vi "Get property names from config.vi"(0 "reference in":refnum<class "metadata.lvclass">, 5 "error in (no error)":errorcluster) -> (10 "section names":string[](array[string]), 14 "reference out":refnum<class "metadata.lvclass">, 15 "nb elements":u16, 16 "Property names []":string[](array[string]), 19 "error out":errorcluster)   [LabVIEW 2019, in "metadata.lvclass"]
uses:
  metadata.lvclass
  <vilib>/Utility/config.llb/NI_LVConfig.lvlib
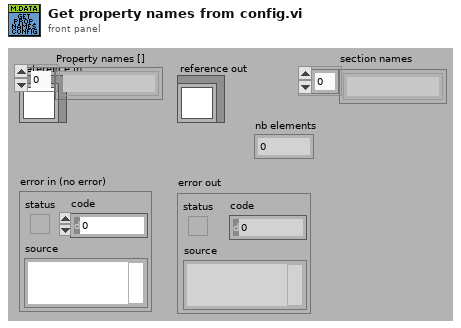
[diagram p1: front panel]
types:
  T1 = typedef "metadata.lvclass/ObjectAttributesRef.ctl" = refnum<data-value>
  T2 = typedef "metadata.lvclass/ObjectAttributes.ctl" = cluster{"MyAttribute":dbl, "System Control":T3, "file info":T4, "Sample info":T5, "Cantilever info":T6, "XYZ piezos":T7, "Mapping":T8, "Fcurve segment":T9[], "Fast fpga segment":T11, "Chirp":T12, "precision (6)":i16, "width (-)":i16, "Metadata":T13, "config filepath":path, "Section names []":string[], "Property names []":string[], "nb elements":u16}
  T3 = typedef "metadata.lvclass/System control parameters.ctl" = cluster{"FPGA SW version":string, "TDMS file version":string, "Instrument":string, "Instrument model":string, "Instrument scanner":string, "Instrument clockrate (Mhz)":string, "Instrument tick time (us)":string}
  T4 = typedef "metadata.lvclass/File info parameters.ctl" = cluster{"Time Stamp":timestamp, "Filename":string, "Filepath":path, "User":string, "Experiment_name":string, "Curve_id":string, "number_segments":u8, "number_consecutive_scans":u32}
  T5 = typedef "metadata.lvclass/Sample info parameters.ctl" = cluster{"Sample name":string, "Sample species":string}
  T6 = typedef "metadata.lvclass/Cantilever info parameters.ctl" = cluster{"spring constant calib method":string, "invOLS calib method":string, "thermal calib deflection channel":string, "model":string, "shape":string, "tip geometry":string, "Laser sum (V)":dbl, "Laser power (mA)":dbl, "invOLS_(nm/V)":dbl, "spring constant nominal (N/m)":dbl, "spring constant calib (N/m)":dbl, "resosnance frequency air calib (Hz)":dbl, "resosnance frequency calib (Hz)":dbl, "quality factor":dbl, "Acoefficident_GCI_(nN.s^1.3/m)":dbl, "half angle (deg)":dbl, "tip radius (m)":dbl, "tip height (m)":dbl, "system mount angle (deg)":dbl}
  T7 = typedef "metadata.lvclass/XYZ piezos parameters.ctl" = cluster{"X stage piezo sensitivity (nm/V)":dbl, "X stage piezo gain":dbl, "X velocity (V/tick)":dbl, "X closed loop":bool, "Y stage piezo sensitivity (nm/V)":dbl, "Y stage piezo gain":dbl, "Y velocity (V/tick)":dbl, "Y closed loop":bool, "Z stage piezo sensitivity (nm/V)":dbl, "Z stage piezo gain":dbl, "Z closed loop":bool, "X position (V)":dbl, "Y position (V)":dbl}
  T8 = typedef "metadata.lvclass/Mapping parameters.ctl" = cluster{"Mapping":bool, "index":u16, "position row":u16, "position column":u16, "next position row":i16, "next position column":i16, "X initial position (V)":dbl, "Y initial position (V)":dbl, "X step size (V)":dbl, "Y step size (V)":dbl}
  T9 = typedef "metadata.lvclass/Fcurve segment.ctl" = cluster{"type":T10, "fast_fpga_trigger":bool, "nb":u8, "duration (ticks)":i64, "nb points":i32, "sampling rate (S/s)":u32, "Zpiezo control out":string, "initial deflection (V)":dbl, "relative setpoint":bool, "setpoint on":bool, "setpoint (V)":dbl, "setpoint trigger channel":string, "velocity (V/tick)":dbl, "Z position setpoint trigger (V)":dbl, "Z retract length (V)":dbl, "dec factor":u32}
  T10 = typedef "metadata.lvclass/Segment type--combobox.ctl" = string
  T11 = typedef "metadata.lvclass/fast fpga segment parameters.ctl" = cluster{"Fast start time trigger":timestamp, "nb_points":u32, "sampling_rate_(S/s)":u32, "duration_(ticks)":u32}
  T12 = typedef "metadata.lvclass/Chirp added parameters.ctl" = cluster{"f start (Hz)":dbl, "f end (Hz)":dbl, "Sweep type":string}
  T13 = typedef "metadata.lvclass/Metadata output --cluster.ctl" = cluster{"Property Names":string[], "Property Values":variant[]}
  T14 = typedef "NI_LVConfig.lvlib/Config Data RefNum.ctl" = refnum<k1>
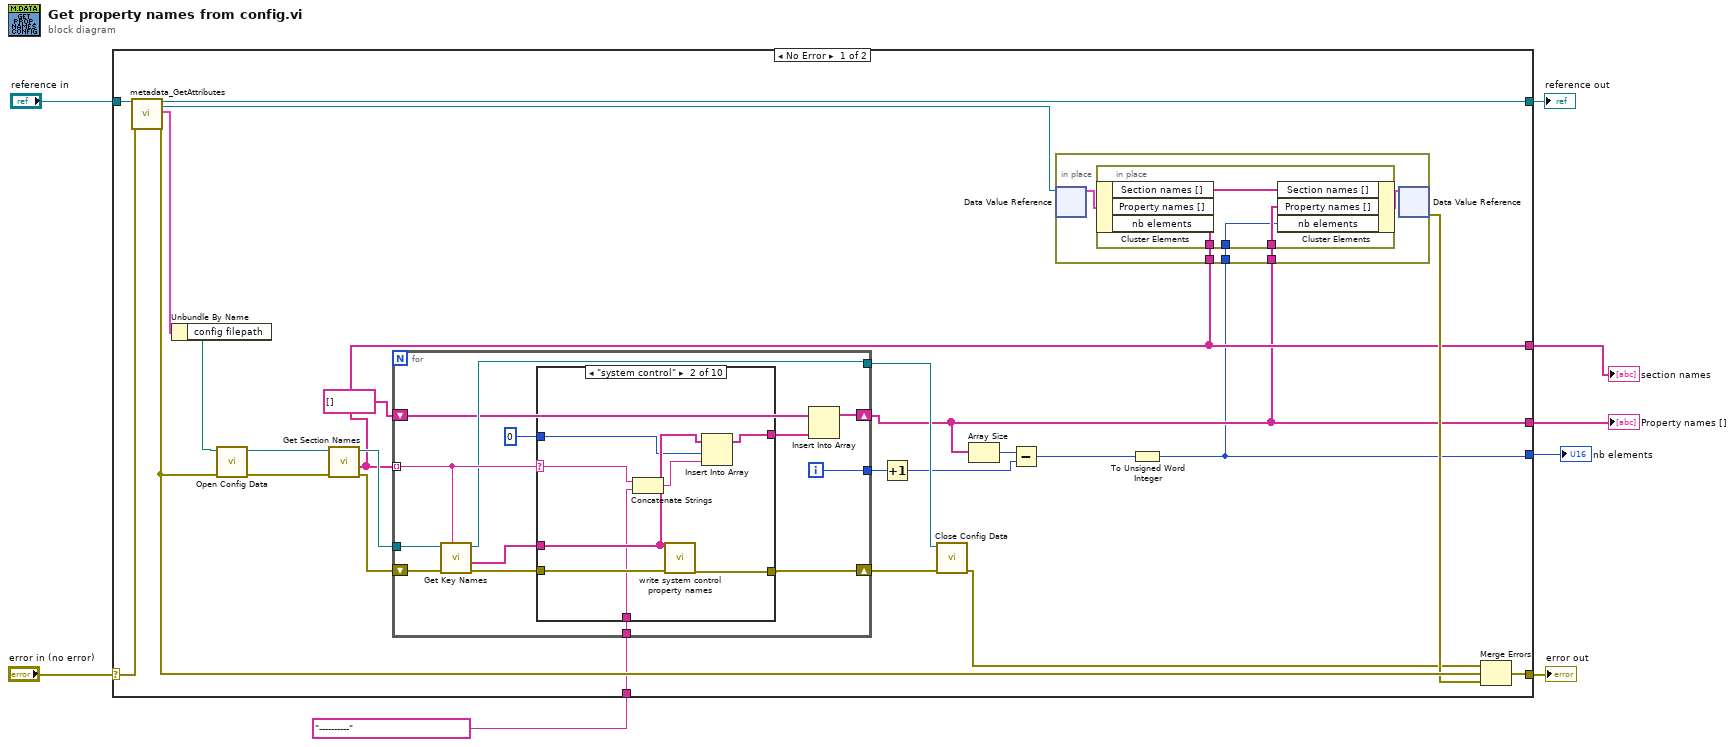
[diagram p0: block diagram]
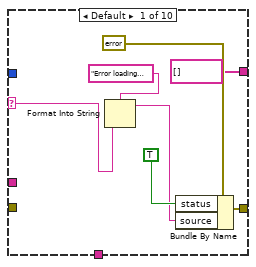
[diagram p2: hidden frame]
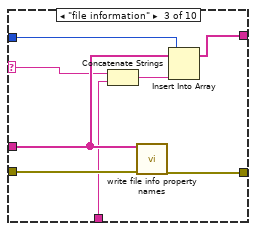
[diagram p3: hidden frame]
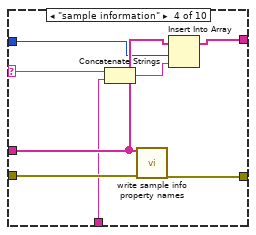
[diagram p4: hidden frame]
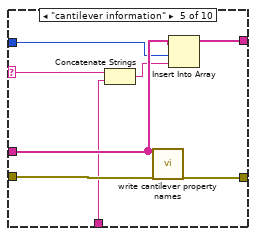
[diagram p5: hidden frame]
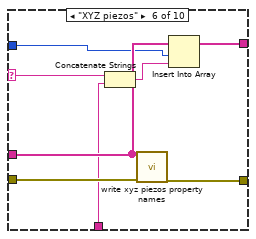
[diagram p6: hidden frame]
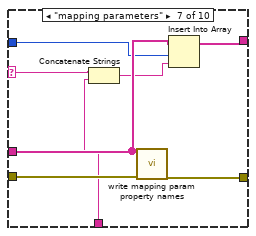
[diagram p7: hidden frame]
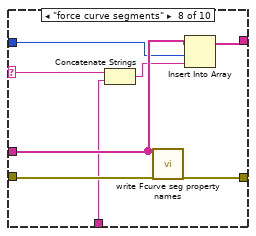
[diagram p8: hidden frame]
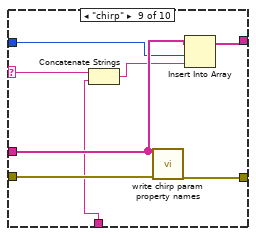
[diagram p9: hidden frame]
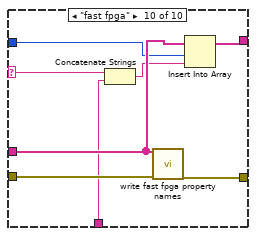
[diagram p10: hidden frame]
diagram:
  n1 = case shown="No Error" "error in (no error)" {
    selector: "error in (no error)" -> [w33 w135]
    tunnel: [w14 w135] -> w7
    tunnel: [w32 w134] -> w5
    tunnel: "reference in" -> [w30 w134]
    tunnel: [w11 _] -> w4
    tunnel: "----------" ("string") -> [w20 _]
    tunnel: [w9 _] -> w2
    tunnel: [w12 _] -> w1
    frame No Error {
      n2 = call "metadata_GetAttributes.vi"("reference in"=w30, "error in (no error)"=w33) -> ("reference out"=w32:refnum<class "metadata.lvclass">, "attributes ref"=w15:T1, "attributes"=w31:T2, "error out"=w21:errorcluster)  [unwired: 14 in]
      n3 = Unbundle By Name(w31) -> ("config filepath"=w29:path)
      n4 = call <vilib>:"Open Config Data.vi"("error in (no error)"=w21, "configuration file path"=w29) -> ("error out"=w27:errorcluster, "refnum"=w28:T14)  [unwired: 7 in, 1 out]
      n5 = call <vilib>:"Get Section Names.vi"("error in (no error)"=w27, "refnum"=w28) -> ("error out"=w25:errorcluster, "section names"=w12:string[], "refnum out"=w26:T14)  [unwired: 7 in]
      n6 = for {
        tunnel: w12 -> [w54] mode=indexing
        tunnel: w26 -> [w53]
        shift-right: [w49] -> w23
        shift-left: w25 -> [w52]
        tunnel: [w48] -> w24
        shift-right: [w46] -> w11
        shift-left: string[] [] ("key names") -> [w47]
        tunnel: w20 -> [w43]
        tunnel: [w42] -> w18
        i -> [w42]
        n7 = call <vilib>:"Get Key Names.vi"("section"=w54, "error in (no error)"=w52, "refnum"=w53) -> ("error out"=w51:errorcluster, "key names"=w50:string[], "refnum out"=w48:T14)  [unwired: 5 in, 1 out]
        n8 = case shown="\"system control\"" w54 {
          selector: w54 -> [w57 w64 w72 w80 w88 w96 w104 w112 w120 w128]
          tunnel: w51 -> [_ w69 w77 w85 w93 w101 w109 w117 w125 w133]
          tunnel: w50 -> [_ w67 w75 w83 w91 w99 w107 w115 w123 w131]
          tunnel: [w60 w68 w76 w84 w92 w100 w108 w116 w124 w132] -> w49
          tunnel: [string[] [] ("key names") w66 w74 w82 w90 w98 w106 w114 w122 w130] -> w45
          tunnel: 0 ("index") -> [_ w65 w73 w81 w89 w97 w105 w113 w121 w129]
          tunnel: w43 -> [_ w62 w71 w78 w86 w94 w102 w111 w118 w126]
          frame Default {
            n9 = Format Into String(format string="Error loading property names sections. Missing Section: \"%s\" in config file!" ("source"), w57) -> (resulting string=w56:string)  [unwired: 2 in, 1 out]
            n10 = Bundle By Name(cluster=errorcluster {"status"=TRUE, "code"=0, "source"="Error loading property names sections. Missing Section in config file!"} ("error out"), "status"=TRUE, "source"=w56) -> (w60:errorcluster)
          }
          frame "system control" {
            n11 = Concatenate Strings(w64, w62) -> (w63:string)
            n12 = call "write system control property names.vi"("Property names.System control"=w67, "error in (no error)"=w69) -> ("error out"=w68:errorcluster)  [unwired: 17 in]
            n13 = Insert Into Array(array=w67, index=w65, new element=w63) -> (w66:string[])
          }
          frame "file information" {
            n14 = Concatenate Strings(w72, w71) -> (w70:string)
            n15 = call "write file info property names.vi"("Property names.File info"=w75, "error in (no error)"=w77) -> ("error out"=w76:errorcluster)  [unwired: 17 in]
            n16 = Insert Into Array(array=w75, index=w73, new element=w70) -> (w74:string[])
          }
          frame "sample information" {
            n17 = Concatenate Strings(w80, w78) -> (w79:string)
            n18 = call "write sample info property names.vi"("Property names.Sample info"=w83, "error in (no error)"=w85) -> ("error out"=w84:errorcluster)  [unwired: 17 in]
            n19 = Insert Into Array(array=w83, index=w81, new element=w79) -> (w82:string[])
          }
          frame "cantilever information" {
            n20 = Concatenate Strings(w88, w86) -> (w87:string)
            n21 = call "write cantilever property names.vi"("Property names.Cantilever calib"=w91, "error in (no error)"=w93) -> ("error out"=w92:errorcluster)  [unwired: 17 in]
            n22 = Insert Into Array(array=w91, index=w89, new element=w87) -> (w90:string[])
          }
          frame "XYZ piezos" {
            n23 = Concatenate Strings(w96, w94) -> (w95:string)
            n24 = call "write xyz piezos property names.vi"("Property names.XYZ piezos"=w99, "error in (no error)"=w101) -> ("error out"=w100:errorcluster)  [unwired: 17 in]
            n25 = Insert Into Array(array=w99, index=w97, new element=w95) -> (w98:string[])
          }
          frame "mapping parameters" {
            n26 = Concatenate Strings(w104, w102) -> (w103:string)
            n27 = call "write mapping param property names.vi"("Property names.Mapping param"=w107, "error in (no error)"=w109) -> ("error out"=w108:errorcluster)  [unwired: 17 in]
            n28 = Insert Into Array(array=w107, index=w105, new element=w103) -> (w106:string[])
          }
          frame "force curve segments" {
            n29 = Concatenate Strings(w112, w111) -> (w110:string)
            n30 = call "write Fcurve seg property names.vi"("Property names.Fcurve Seg"=w115, "error in (no error)"=w117) -> ("error out"=w116:errorcluster)  [unwired: 17 in]
            n31 = Insert Into Array(array=w115, index=w113, new element=w110) -> (w114:string[])
          }
          frame "chirp" {
            n32 = Concatenate Strings(w120, w118) -> (w119:string)
            n33 = call "write chirp param property names.vi"("Property names.Chirp Param"=w123, "error in (no error)"=w125) -> ("error out"=w124:errorcluster)  [unwired: 17 in]
            n34 = Insert Into Array(array=w123, index=w121, new element=w119) -> (w122:string[])
          }
          frame "fast fpga" {
            n35 = Concatenate Strings(w128, w126) -> (w127:string)
            n36 = call "write fast fpga property names.vi"("Property names.Fast fpga param"=w131, "error in (no error)"=w133) -> ("error out"=w132:errorcluster)  [unwired: 17 in]
            n37 = Insert Into Array(array=w131, index=w129, new element=w127) -> (w130:string[])
          }
        }
        n38 = Insert Into Array(array=w47, new element=w45) -> (w46:string[])  [unwired: 1 in]
      }
      n39 = Increment(x=w18) -> (x+1=w17:i32)
      n40 = call <vilib>:"Close Config Data.vi"("error in (no error)"=w23, "refnum"=w24) -> ("error out"=w13:errorcluster)  [unwired: 8 in, 1 out]
      n41 = Array Size(array=w11) -> (size(s)=w19:i32)
      n42 = Subtract(x=w19, y=w17) -> (x-y=w10:i32)
      n43 = To Unsigned Word Integer(number=w10) -> (unsigned 16bit integer=w9:u16)
      n44 = in-place {
        in-place-border: w12 -> [w36]
        in-place-border: w11 -> [w35]
        in-place-border: w9 -> [w34]
        n45 = in-place-dvr #1(w15) -> (w37:T2)  [unwired: 1 out]
        n46 = in-place {
          in-place-border: w36 -> [w41]
          in-place-border: w35 -> [w40]
          in-place-border: w34 -> [w39]
          n47 = in-place-cluster #2(w37) -> ()  [unwired: 3 out]
          n48 = in-place-cluster #2("Section names []"=w41, "Property names []"=w40, "nb elements"=w39) -> (w38:T2)
        }
        n49 = in-place-dvr #1(w38) -> (w16:errorcluster)  [unwired: 1 out]
      }
      n50 = Merge Errors(w13, w21, w16) -> (w14:errorcluster)
    }
    frame Error {
    }
  }
  "error out" <- w7
  "reference out" <- w5
  "Property names []" <- w4
  "nb elements" <- w2
  "section names" <- w1
